vi "Create Protection and Rolling Counter Addon.vi"(7 "Configuration (.dat)":path, 8 "error in (no error)":errorcluster, 9 "Port":string, 10 "Name":string, 11 "Custom Devices Ref in":refnum<k24>) -> (0 "error out":errorcluster, 3 "Custom Devices Ref":refnum<k24>)   [LabVIEW 2025, in "Protection and Counter Addon System Definition API.lvlib"]
uses:
  Protection and Counter Addon System Definition API.lvlib
  NationalInstruments.VeriStand.SystemDefinitionAPI
  Addon/Addon Shared/SubVIs/GUID Lookup.vi
  <vilib>/NI/NI VeriStand Advanced SysDef API/_SubVIs/SysDef.Property.Get.String.vi
  <vilib>/NI/NI VeriStand Custom Device Import and Export Tool/ImportExport.lvlib
  Addon/Addon Shared/Protection and Counter Addon Shared.lvlib
  <vilib>/NI/NI VeriStand Advanced SysDef API/SysDef API/Advanced System Definition.lvlib
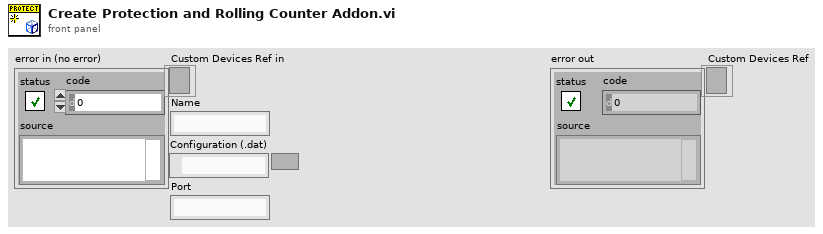
[diagram p1: front panel]
types:
  T1 = typedef "Custom Device API.lvlib/Custom Device Item Ref.ctl" = u64
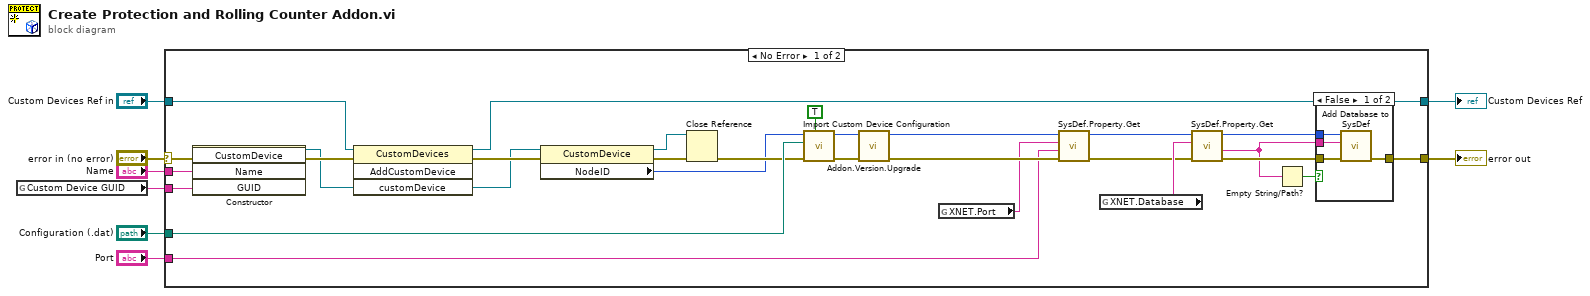
[diagram p0: block diagram]
diagram:
  n1 = global read "GUID Lookup.vi" "Custom Device GUID"() -> (w2:string)
  n2 = case shown="No Error" "error in (no error)" {
    selector: "error in (no error)" -> [w34 w43]
    tunnel: w2 -> [w36 _]
    tunnel: [w17 w43] -> w8
    tunnel: "Custom Devices Ref in" -> [w35 w42]
    tunnel: [w26 w42] -> w6
    tunnel: "Name" -> [w28 _]
    tunnel: "Configuration (.dat)" -> [w27 _]
    tunnel: "Port" -> [w9 _]
    frame No Error {
      n3 = constructor class="CustomDevice"(error in=w34, "Name"=w28, "GUID"=w36) -> (reference out=w29:refnum<k24>, error out=w30:errorcluster)  [unwired: 2 in, 3 out]
      n4 = invoke class="CustomDevices" method="AddCustomDevice"(reference=w35, error in=w30, "customDevice"=w29) -> (reference out=w26:refnum<k24>, error out=w33:errorcluster)  [unwired: 1 in, 2 out]
      n5 = property class="CustomDevice"(reference=w29, error in=w33) -> (reference out=w31:refnum<k24>, error out=w32:errorcluster, "NodeID"=w24:u64)
      n6 = Close Reference(reference=w31, error in (no error)=w32) -> (error out=w25:errorcluster)
      n7 = call <vilib>:"Import Custom Device Configuration.vi"("Overwrite Existing?"=TRUE, "error in (no error)"=w25, "Path"=w27, "NodeID"=w24) -> ("error out"=w21:errorcluster, "NodeID out"=w22:u64)  [unwired: 5 in, 1 out]
      n8 = call "Addon.Version.Upgrade.vi"("error in (no error)"=w21, "Device Item Ref in in"=w22) -> ("error out"=w11:errorcluster, "Device Item Ref out"=w14:T1)  [unwired: 8 in]
      n9 = global read "GUID Lookup.vi" "XNET.Port"() -> (w10:string)
      n10 = call-poly <vilib>:"SysDef.Property.Get.vi"("error in (no error)"=w11, "Value"=w9, "Property Name"=w10, "nodeID"=w14) -> ("error out"=w12:errorcluster, "nodeID out"=w13:u64)  [unwired: 4 in, 2 out]
      n11 = global read "GUID Lookup.vi" "XNET.Database"() -> (w20:string)
      n12 = call-poly <vilib>:"SysDef.Property.Get.vi"("error in (no error)"=w12, "Property Name"=w20, "nodeID"=w13) -> ("error out"=w18:errorcluster, "Value out"=w16:string, "nodeID out"=w19:u64)  [unwired: 5 in, 1 out]
      n13 = Empty String/Path?(string/path=w16) -> (empty?=w15:bool)
      n14 = case shown="False" w15 {
        tunnel: w19 -> [w40 _]
        tunnel: w18 -> [w39 w41]
        tunnel: [w38 w41] -> w17
        tunnel: w16 -> [w37 _]
        frame False {
          n15 = call "Add Database to SysDef.vi"("error in"=w39, "DB Alias"=w37, "Item Ref in"=w40) -> ("error out"=w38:errorcluster)  [unwired: 7 in, 1 out]
        }
        frame True {
        }
      }
    }
    frame Error {
    }
  }
  "error out" <- w8
  "Custom Devices Ref" <- w6
